vi "Save_reference_Raw_data.vi"(6 "Data_struct":refnum<k24>[](array[refnum]), 7 "chkeach_ch":bool, 8 "错误输入（无错误）":errorcluster, 9 "Ref_monitordata_struct":refnum<k24>[](array[refnum]), 10 "Refdata_struct":refnum<k24>[](array[refnum]), 11 "ILSTS":refnum<k24>) -> (0 "错误输出":errorcluster)   [LabVIEW 2017]
doc: "Save reference Raw data"
uses:
  D:/test/ILSTS/LV_IL_Sample/DLL/STSProcess.dll
  DLL/STSProcess.dll
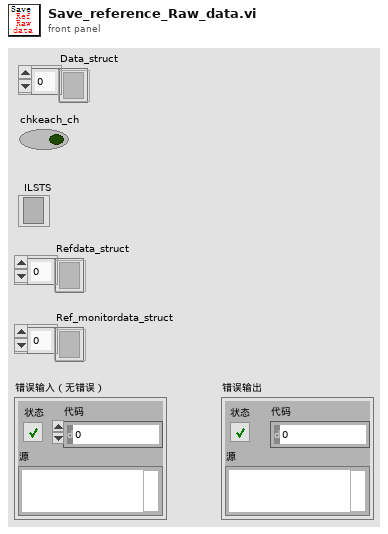
[diagram p1: front panel]
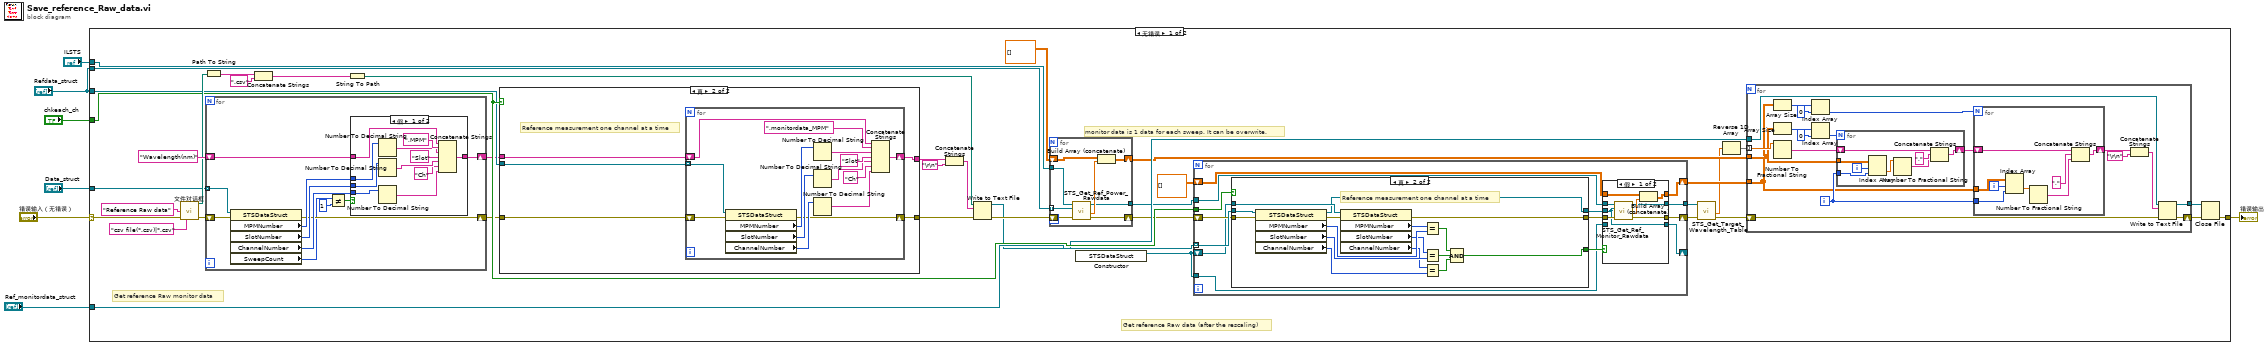
[diagram p0: block diagram]
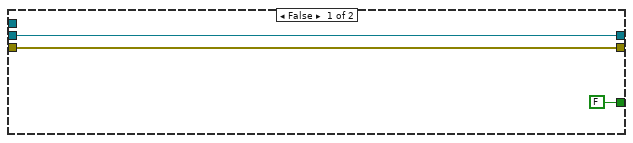
[diagram p3: hidden frame]
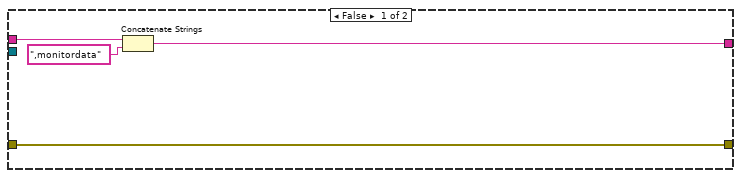
[diagram p4: hidden frame]
diagram:
  n1 = case shown="无错误" "错误输入（无错误）" {
    selector: "错误输入（无错误）" -> [w33 w181]
    tunnel: [w20 w181] -> w7
    tunnel: "Ref_monitordata_struct" -> [w46 _]
    tunnel: "chkeach_ch" -> [w30 _]
    tunnel: "ILSTS" -> [w45 _]
    tunnel: "Refdata_struct" -> [w44 _]
    tunnel: "Data_struct" -> [w31 _]
    tunnel: "Refdata_struct" -> [w29 _]
    frame No Error {
      # "Get reference Raw monitor data"
      # "monitor data is 1 data for each sweep. It can be overwrite."
      # "Get reference Raw data (after the rescaling)"
      n2 = call "文件对话框"("default name"="Reference Raw data" ("字符串"), "error in"=w33, "pattern (all files)"="csv file(*.csv)|*.csv") -> ("selected path"=w37:path, "error out"=w38:errorcluster)  [unwired: 9 in, 2 out]
      n3 = Path To String(path=w37) -> (string=w24:string)
      n4 = for {
        tunnel: w31 -> [w168] mode=indexing
        shift-right: [w162] -> w28
        shift-left: "Wavelength(nm)" -> [w163]
        shift-right: [w161] -> w27
        shift-left: w38 -> [w167]
        n5 = property on="属性节点" class="STSDataStruct"(reference=w168, error in=w167) -> (error out=w161:errorcluster, "MPMNumber"=w164:i32, "SlotNumber"=w165:i32, "ChannelNumber"=w166:i32, "SweepCount"=w160:i32)  [unwired: 1 out]
        n6 = Not Equal?(x=w160, y=1) -> (x != y?=w158:bool)
        n7 = case shown="假" w158 {
          tunnel: w166 -> [w179 _]
          tunnel: w165 -> [w178 _]
          tunnel: w164 -> [w177 _]
          tunnel: w163 -> [w176 w180]
          tunnel: [w169 w180] -> w162
          frame False {
            n8 = Number To Decimal String(number=w177) -> (decimal integer string=w174:string)  [unwired: 1 in]
            n9 = Number To Decimal String(number=w178) -> (decimal integer string=w172:string)  [unwired: 1 in]
            n10 = Number To Decimal String(number=w179) -> (decimal integer string=w170:string)  [unwired: 1 in]
            n11 = Concatenate Strings(w176, ",MPM" ("字符串"), w174, "Slot" ("字符串"), w172, "Ch" ("字符串"), w170) -> (w169:string)
          }
          frame True {
          }
        }
      }
      n12 = Concatenate Strings(w24, ".csv" ("名称或相对路径")) -> (w35:string)
      n13 = String To Path(string=w35) -> (path=w34:path)
      n14 = case shown="真" w30 {
        tunnel: w29 -> [_ w142]
        tunnel: w28 -> [w138 w141]
        tunnel: w27 -> [w135 w143]
        tunnel: [w136 w140] -> w26
        tunnel: [w135 w139] -> w25
        frame False {
          n15 = Concatenate Strings(w138, ",monitordata" ("字符串")) -> (w136:string)
        }
        frame True {
          # "Reference measurement one channel at a time"
          n16 = for {
            tunnel: w142 -> [w157] mode=indexing
            shift-right: [w145] -> w140
            shift-left: w141 -> [w152]
            shift-right: [w144] -> w139
            shift-left: w143 -> [w156]
            n17 = property on="属性节点" class="STSDataStruct"(reference=w157, error in=w156) -> (error out=w144:errorcluster, "MPMNumber"=w153:i32, "SlotNumber"=w154:i32, "ChannelNumber"=w155:i32)  [unwired: 1 out]
            n18 = Number To Decimal String(number=w153) -> (decimal integer string=w150:string)  [unwired: 1 in]
            n19 = Number To Decimal String(number=w154) -> (decimal integer string=w148:string)  [unwired: 1 in]
            n20 = Number To Decimal String(number=w155) -> (decimal integer string=w146:string)  [unwired: 1 in]
            n21 = Concatenate Strings(w152, ",monitordata_MPM" ("字符串"), w150, "Slot" ("字符串"), w148, "Ch" ("字符串"), w146) -> (w145:string)
          }
        }
      }
      n22 = Concatenate Strings(w26, "\r\n") -> (w41:string)
      n23 = Write to Text File(file (use dialog)=w34, text=w41, error in=w25) -> (refnum out=w23:refnum<file>, error out=w32:errorcluster)  [unwired: 1 in, 1 out]
      n24 = for {
        tunnel: w44 -> [w133] mode=indexing
        tunnel: w45 -> [w134]
        shift-right: [w128] -> w18
        shift-left: w32 -> [w132]
        shift-right: [w130] -> w11
        shift-left: sgl[][] [] -> [w129]
        tunnel: [w127] -> w17
        n25 = call "STS_Get_Ref_Power_Rawdata.vi"("错误输入（无错误）"=w132, "setting"=w133, ".NET引用句柄输入"=w134) -> ("error out"=w128:errorcluster, "powerdata"=w131:sgl[], "引用输出"=w127:refnum<k24>)  [unwired: 6 in]
        n26 = Build Array (concatenate)(w129, w131) -> (w130:sgl[][])
      }
      n27 = constructor class="STSDataStruct"() -> (reference out=w8:refnum<k24>)  [unwired: 3 in, 2 out]
      n28 = for {
        tunnel: w30 -> [w95]
        tunnel: w46 -> [w94] mode=indexing
        shift-right: [w86] -> w14
        shift-left: w18 -> [w93]
        shift-right: [w83] -> _
        shift-left: w8 -> [w92]
        tunnel: w17 -> [w89]
        shift-right: [w88] -> w12
        shift-left: sgl[][] [] -> [w87]
        tunnel: [w85] -> w15
        tunnel: w8 -> [w82]
        n29 = case shown="真" w95 {
          tunnel: w94 -> [w108 w126]
          tunnel: w93 -> [w109 w125]
          tunnel: w92 -> [_ w124]
          tunnel: [FALSE w113] -> w91
          tunnel: [w109 w112] -> w90
          tunnel: [w108 w111] -> w84
          frame False {
          }
          frame True {
            # "Reference measurement one channel at a time"
            n30 = property on="属性节点" class="STSDataStruct"(reference=w126, error in=w125) -> (reference out=w111:refnum<k24>, error out=w123:errorcluster, "MPMNumber"=w121:i32, "SlotNumber"=w119:i32, "ChannelNumber"=w118:i32)
            n31 = property class="STSDataStruct"(reference=w124, error in=w123) -> (error out=w112:errorcluster, "MPMNumber"=w122:i32, "SlotNumber"=w120:i32, "ChannelNumber"=w117:i32)  [unwired: 1 out]
            n32 = Equal?(x=w122, y=w121) -> (x = y?=w116:bool)
            n33 = Equal?(x=w120, y=w119) -> (x = y?=w115:bool)
            n34 = Equal?(x=w117, y=w118) -> (x = y?=w114:bool)
            n35 = Compound Arithmetic op=AND ("复合运算")(w116, w115, w114) -> (w113:bool)
          }
        }
        n36 = case shown="假" w91 {
          tunnel: w90 -> [w103 w106]
          tunnel: w84 -> [w96 _]
          tunnel: w89 -> [w102 w105]
          tunnel: [w100 w107] -> w88
          tunnel: w87 -> [w99 w107]
          tunnel: [w98 w106] -> w86
          tunnel: [w97 w105] -> w85
          tunnel: [w96 w104] -> w83
          tunnel: w82 -> [_ w104]
          frame False {
            n37 = call "STS_Get_Ref_Monitor_Rawdata.vi"("错误输入（无错误）"=w103, "setting"=w96, ".NET引用句柄输入"=w102) -> ("error out"=w98:errorcluster, "monitordata"=w101:sgl[], "引用输出"=w97:refnum<k24>)  [unwired: 6 in]
            n38 = Build Array (concatenate)(w99, w101) -> (w100:sgl[][])
          }
          frame True {
          }
        }
      }
      n39 = call "STS_Get_Target_Wavelength_Table.vi"("错误输入（无错误）"=w14, ".NET引用句柄输入"=w15) -> ("error out"=w13:errorcluster, "wavelengths"=w10:dbl[])  [unwired: 7 in, 1 out]
      n40 = Reverse 1D Array(array=w10) -> (reversed array=w9:dbl[])
      n41 = for {
        tunnel: w9 -> [w65] mode=indexing
        tunnel: w12 -> [w48]
        tunnel: w23 -> [w57]
        tunnel: [w56] -> w22
        tunnel: w11 -> [w55]
        shift-right: [w62] -> w21
        shift-left: w13 -> [w63]
        i -> [w51]
        n42 = Array Size(array=w48) -> (size(s)=w50:i32[])
        n43 = Array Size(array=w55) -> (size(s)=w60:i32[])
        n44 = Number To Fractional String(number=w65) -> (F-format string=w64:string)  [unwired: 3 in]
        n45 = Index Array(array=w50, index=0 ("索引")) -> (element=w47:i32)
        n46 = Index Array(array=w60, index=0 ("索引")) -> (element=w58:i32)
        n47 = for {
          N: w58 -> [_]
          tunnel: w55 -> [w81]
          tunnel: w51 -> [w80]
          shift-right: [w76] -> w53
          shift-left: w64 -> [w77]
          i -> [w79]
          n48 = Index Array(array=w81, index (row)=w79, index (col)=w80) -> (element=w78:sgl)
          n49 = Number To Fractional String(number=w78) -> (F-format string=w74:string)  [unwired: 3 in]
          n50 = Concatenate Strings(w77, "," ("字符串"), w74) -> (w76:string)
        }
        n51 = for {
          N: w47 -> [_]
          tunnel: w48 -> [w73]
          tunnel: w51 -> [w72]
          shift-right: [w68] -> w52
          shift-left: w53 -> [w69]
          i -> [w71]
          n52 = Index Array(array=w73, index (row)=w71, index (col)=w72) -> (element=w70:sgl)
          n53 = Number To Fractional String(number=w70) -> (F-format string=w66:string)  [unwired: 3 in]
          n54 = Concatenate Strings(w69, "," ("字符串"), w66) -> (w68:string)
        }
        n55 = Concatenate Strings(w52, "\r\n") -> (w61:string)
        n56 = Write to Text File(file (use dialog)=w57, text=w61, error in=w63) -> (refnum out=w56:refnum<file>, error out=w62:errorcluster)  [unwired: 1 in, 1 out]
      }
      n57 = Close File(refnum=w22, error in=w21) -> (error out=w20:errorcluster)  [unwired: 1 out]
    }
    frame Error {
    }
  }
  "错误输出" <- w7
